vi "LoadTypeCache.vi"(8 "error in (no error)":errorcluster, 11 "Any HDF5 Refnum":T1) -> (0 "error out":errorcluster, 2 "# Types Loaded":i32, 3 "Any HDF5 Refnum out":T1)   [LabVIEW 2017]
uses:
  <vilib>/UPVI/lvhdf5/library.llb/HDF5 Ref.ctl
  <vilib>/UPVI/lvhdf5/datatype.llb/private/LVTypeElement.ctl
  <vilib>/Utility/VariantDataType/UnitInfo.ctl
  <vilib>/Utility/VariantDataType/UnitType.ctl
  <vilib>/UPVI/lvhdf5/group.llb/H5G_obj_t.ctl
  <vilib>/Utility/VariantDataType/VariantType.lvlib
panel:
  in  "LVTypeElement":T2 {"TD" format="%.0x"}
  # "LVHDF5 Toolkit\nCopyright (c) 2005-2013 by Jason D. Sommerville\nCopyright (c) 2014 by UPVI, LLC.\n\nThis use and distribution of this file is governed by the terms found in \nLICENSE.txt distributed with this toolkit and installed at\n <user.lib>\\_lvhdf5\\LICENSE.txt"
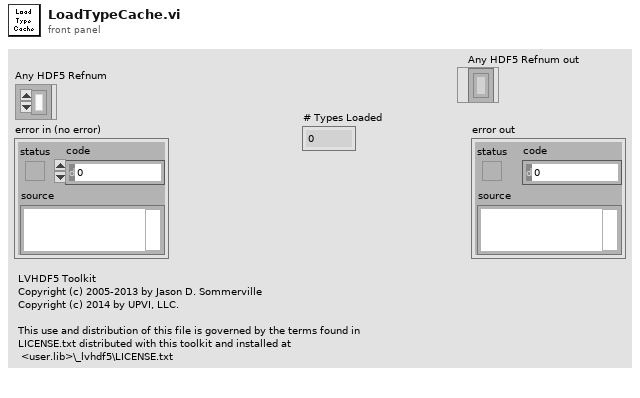
[diagram p1: front panel]
types:
  T1 = typedef "HDF5 Ref.ctl" = refnum<k1>
  T2 = typedef "LVTypeElement.ctl" = cluster{"Name":string, "TD":i16[], "Type Ref":T1, "Description":string, "Unit String":string, "Units":T3[], "Status":cluster{"MustCommit":bool, "IsCommitted":bool}}
  T3 = typedef "VariantType.lvlib/UnitInfo.ctl" = cluster{"UnitType":T4, "Exponent":i16}
  T4 = typedef "VariantType.lvlib/UnitType.ctl" = enum16{"Radians", "Steradians", "Seconds", "Meters", "Kilograms", "Amperes", "Kelvins", "Moles", "Candelas", "InvalidUnit"}
  T5 = enum16{"find by lvtype", "find by h5type", "index", "push", "pop", "delete last", "dequeue", "delete all"}
  T6 = typedef "H5G_obj_t.ctl" = i32
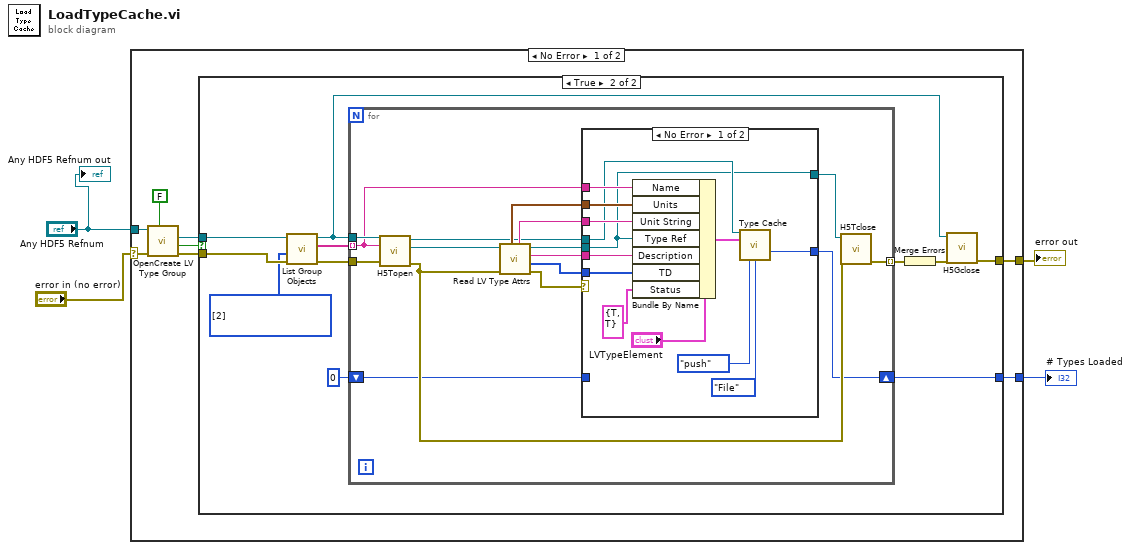
[diagram p0: block diagram]
diagram:
  n1 = case shown="No Error" "error in (no error)" {
    selector: "error in (no error)" -> [w6 w56]
    tunnel: [w8 w56] -> w4
    tunnel: "Any HDF5 Refnum" -> [w7 _]
    tunnel: [w5 _] -> w1
    frame No Error {
      n2 = call <vilib>:"OpenCreate LV Type Group.vi"("Create if not found (F)"=FALSE, "error in (no error)"=w6, "Any HDF5 Refnum"=w7) -> ("error out"=w10:errorcluster, "Opened?"=w11:bool, "LVHDF5 Type Group"=w9:T1)  [unwired: 3 in, 1 out]
      n3 = case shown="True" w11 {
        tunnel: w10 -> [w13 w23]
        tunnel: w9 -> [_ w24]
        tunnel: [w13 w17] -> w8
        tunnel: [_ w15] -> w5
        frame False {
        }
        frame True {
          w14 = T6[] [2] items=["H5G_UNKNOWN"=-1, "H5G_GROUP"=0, "H5G_DATASET"=1, "H5G_TYPE"=2, "H5G_LINK"=3, "H5G_UDLINK"=4] ("Object Types (any)")
          n4 = call <vilib>:"List Group Objects.vi"("error in (no error)"=w23, "Object Types (any)"=w14, "HDF5 Loc Ref"=w24) -> ("error out"=w21:errorcluster, "Object Names"=w22:string[], "HDF5 Loc Ref out"=w18:T1)  [unwired: 3 in, 1 out]
          n5 = for {
            tunnel: w18 -> [w39]
            tunnel: w22 -> [w34] mode=indexing
            tunnel: w21 -> [w40]
            tunnel: [w29] -> w20 mode=indexing
            shift-right: [w28] -> w15
            shift-left: 0 ("Count") -> [w27]
            n6 = call <vilib>:"H5Topen.vi"("error in (no error)"=w40, "name"=w34, "HDF5 Location"=w39) -> ("error out"=w31:errorcluster, "HDF5 Type Ref"=w38:T1, "HDF5 Location out"=w32:T1)  [unwired: 4 in]
            n7 = call <vilib>:"Read LV Type Attrs.vi"("error in (no error)"=w31, "LVType Ref"=w38) -> ("error out"=w25:errorcluster, "Type Descriptor"=w26:i16[], "Type Name"=w35:string, "LVType Ref out"=w33:T1, "Unit String"=w37:string, "Units"=w36:T3[])  [unwired: 4 in]
            n8 = case shown="No Error" w25 {
              tunnel: w32 -> [w45 _]
              tunnel: w37 -> [w50 _]
              tunnel: w36 -> [w51 _]
              tunnel: w35 -> [w49 _]
              tunnel: w34 -> [w52 _]
              tunnel: w33 -> [w44 w55]
              tunnel: w26 -> [w48 _]
              tunnel: [w44 w55] -> w30
              tunnel: [w43 w54] -> w28
              tunnel: w27 -> [_ w54]
              frame No Error {
                n9 = Bundle By Name(cluster="LVTypeElement", "Name"=w52, "Units"=w51, "Unit String"=w50, "Type Ref"=w44, "Description"=w49, "TD"=w48, "Status"=cluster{"MustCommit":bool, "IsCommitted":bool} {"MustCommit"=TRUE, "IsCommitted"=TRUE}) -> (w47:T2)
                n10 = call <vilib>:"Type Cache.vi"("HDF5  Loc Ref"=w45, "LVTypeElement in"=w47, "operation"=T5."push", "Type"=enum16{"File", "Memory"}."File") -> ("Count"=w43:i32)  [unwired: 8 in, 3 out]
              }
              frame Error {
              }
            }
            n11 = call <vilib>:"H5Tclose.vi"("error in (no error)"=w31, "HDF5 Datatype Ref"=w30) -> ("error out"=w29:errorcluster)  [unwired: 7 in]
          }
          n12 = Merge Errors(w20) -> (w19:errorcluster)
          n13 = call <vilib>:"H5Gclose.vi"("error in (no error)"=w19, "HDF5 Group Ref"=w18) -> ("error out"=w17:errorcluster)  [unwired: 7 in]
        }
      }
    }
    frame Error {
    }
  }
  "error out" <- w4
  "# Types Loaded" <- w1
  "Any HDF5 Refnum out" <- "Any HDF5 Refnum"
